vi "LFA_Stop.vi"(8 "error in (no error)":errorcluster, 11 "LightField Automation in":refnum<class "LightField Automation.lvclass">) -> (0 "error out":errorcluster, 3 "LightField Automation out":refnum<class "LightField Automation.lvclass">)   [LabVIEW 2013, in "LightField Automation.lvclass"]
uses:
  LightField Automation.lvclass
  LightField Automation.lvclass/LightField Automation.ctl
  C:/Program Files/Princeton Instruments/LightField/AddInViews/PrincetonInstruments.LightFieldViewV3.dll
  Program Files/Princeton Instruments/LightField/AddInViews/PrincetonInstruments.LightFieldViewV3.dll
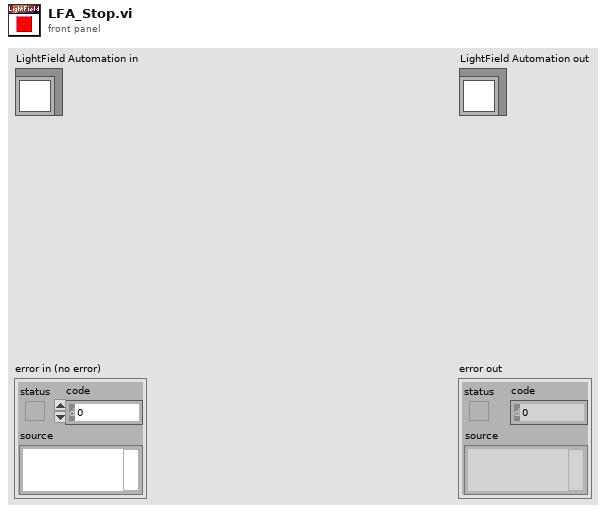
[diagram p1: front panel]
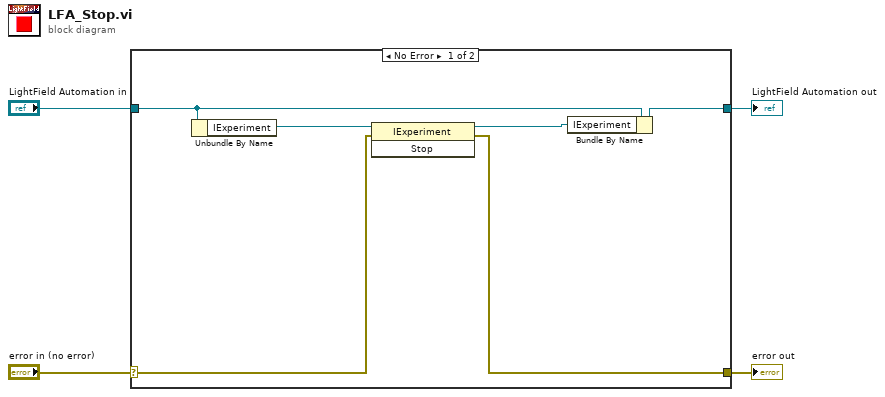
[diagram p0: block diagram]
diagram:
  n1 = case shown="No Error" "error in (no error)" {
    selector: "error in (no error)" -> [w6 w12]
    tunnel: [w5 w12] -> w3
    tunnel: [w9 w11] -> w1
    tunnel: "LightField Automation in" -> [w10 w11]
    frame No Error {
      n2 = Unbundle By Name(w10) -> ("IExperiment"=w8:refnum<k24>)
      n3 = invoke class="IExperiment" method="Stop"(reference=w8, error in=w6) -> (reference out=w7:refnum<k24>, error out=w5:errorcluster)  [unwired: 1 in, 1 out]
      n4 = Bundle By Name(cluster=w10, "IExperiment"=w7) -> (w9:refnum<class "LightField Automation.lvclass">)
    }
    frame Error {
    }
  }
  "error out" <- w3
  "LightField Automation out" <- w1
